vi "get_value_for_string.vi"(8 "error in (no error)":errorcluster, 11 "Value in":refnum<class "Value.lvclass">) -> (0 "error out":errorcluster, 3 "string_value":string)   [LabVIEW 2020, in "toml_edit.lvlib" / "Value.lvclass"]
uses:
  Value.lvclass
  value_type--enum.ctl
  Value.lvclass/Value.ctl
  dragon_toml_64.dll
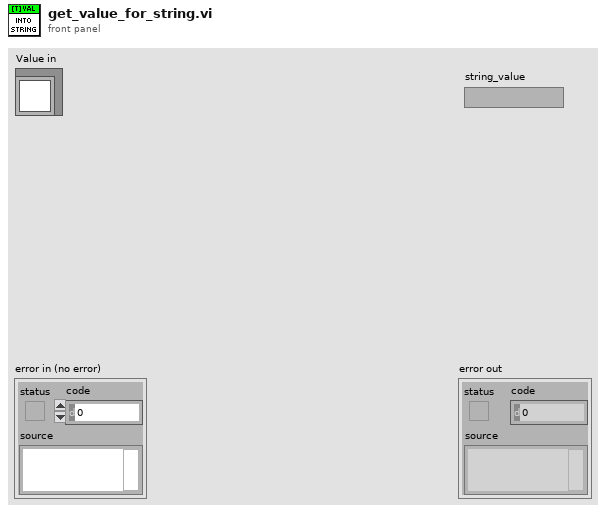
[diagram p1: front panel]
types:
  T1 = typedef "toml_edit.lvlib/Value.lvclass/value_type--enum.ctl" = enum16{"Unknown", "String", "Integer", "Float", "Boolean", "Datetime", "Array", "InlineTable"}
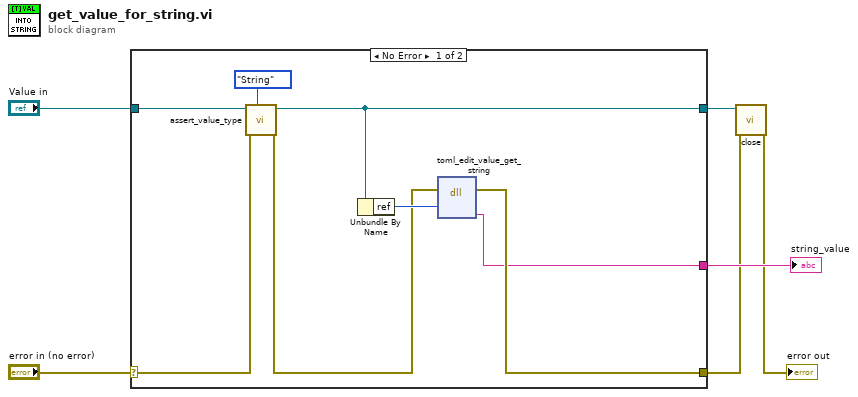
[diagram p0: block diagram]
diagram:
  n1 = case shown="No Error" "error in (no error)" {
    selector: "error in (no error)" -> [w10 w15]
    tunnel: "Value in" -> [w11 w16]
    tunnel: [w7 _] -> w4
    tunnel: [w14 w15] -> w3
    tunnel: [w8 w16] -> w2
    frame No Error {
      n2 = call "assert_value_type.vi"("value_type"=value_type--enum."String", "error in (no error)"=w10, "Value in"=w11) -> ("error out"=w9:errorcluster, "Value out"=w8:refnum<class "Value.lvclass">)  [unwired: 7 in]
      n3 = Unbundle By Name(w8) -> ("ref"=w13:u64)
      n4 = dll-call lib="C:/Users/JamesMcNally/Documents/toml-edit-labview/lv_src/dragon_toml_*.*" fn="toml_edit_value_get_string"(error in=w9, "item_ref"=w13) -> (error out=w14:errorcluster, "value_string"=w7:string)  [unwired: 5 in, 1 out]
    }
    frame Error {
    }
  }
  "string_value" <- w4
  n5 = call "close.vi"("error in (no error)"=w3, "Value in"=w2) -> ("error out"=→"error out":errorcluster)  [unwired: 9 in]
